vi "Get Manager.vi"(8 "error in (no error)":errorcluster, 11 "Message in":refnum<class "Message.lvclass">) -> (0 "error out":errorcluster, 2 "Manager":refnum<class "Manager.lvclass">, 3 "Message out":refnum<class "Message.lvclass">)   [LabVIEW 2020, in "Stream-Simple-Msg.lvlib" / "Message.lvclass"]
uses:
  Message.lvclass
  Manager/Manager.lvclass
  Message.lvclass/Message.ctl
  Endpoint/Endpoint.lvclass
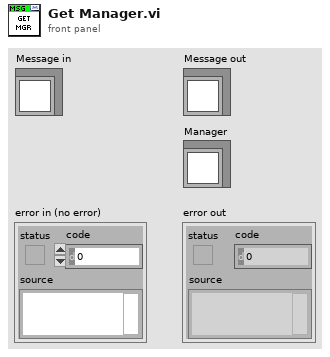
[diagram p1: front panel]
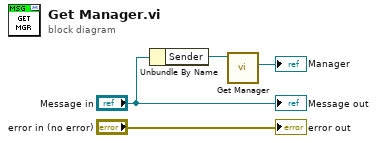
[diagram p0: block diagram]
diagram:
  n1 = Unbundle By Name("Message in") -> ("Sender"=w2:refnum<class "Endpoint.lvclass">)
  n2 = call "Get Manager.vi"("Endpoint in"=w2) -> ("Manager"=→"Manager":refnum<class "Manager.lvclass">)  [unwired: 8 in, 2 out]
  "error out" <- "error in (no error)"
  "Message out" <- "Message in"
